vi "Konversi_Case Structure.vi"() -> ()   [LabVIEW 2020]
panel:
  in  "Case":i32
  in  "stop 2":bool
  out "Fahrenheit":dbl(slide) scale=32.0..212.0
  out "Kelvin":dbl(slide) scale=273.0..373.0
  out "Reamur":dbl(slide) scale=0.0..80.0
  in  "Celcius":dbl(slide) scale=0.0..100.0
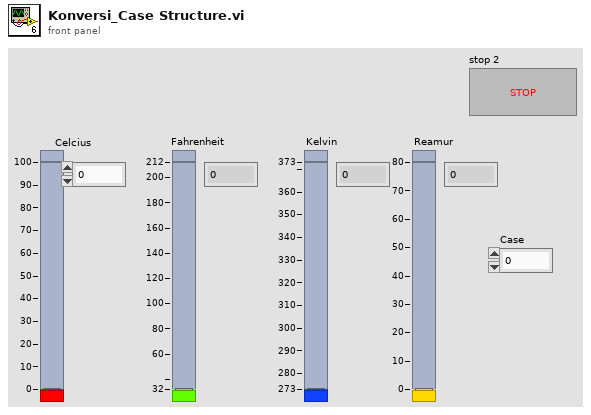
[diagram p1: front panel]
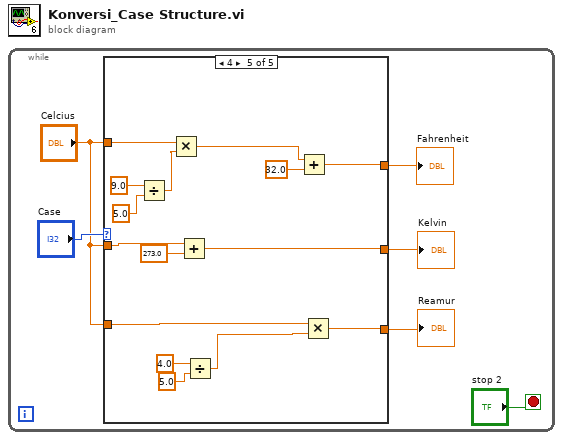
[diagram p0: block diagram]
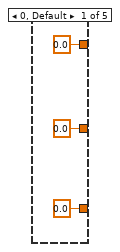
[diagram p2: hidden frame]
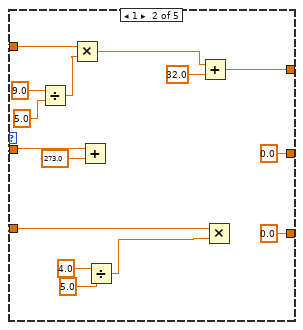
[diagram p3: hidden frame]
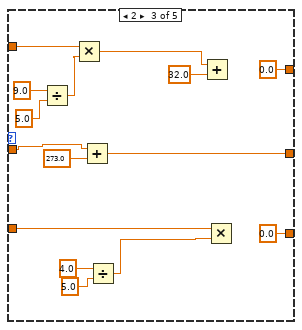
[diagram p4: hidden frame]
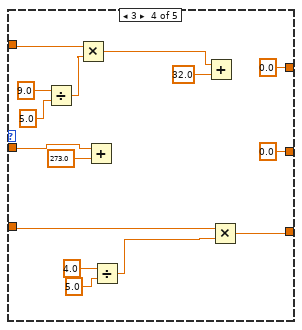
[diagram p5: hidden frame]
diagram:
  n1 = while {
    stop <- "stop 2" stop-if-true
    n2 = case shown="4" "Case" {
      tunnel: [0.0 w17 0.0 0.0 w58] -> w5
      tunnel: [0.0 0.0 w26 0.0 w57] -> w4
      tunnel: "Celcius" -> [_ w15 w29 w44 w59]
      tunnel: [0.0 0.0 0.0 w42 w56] -> w3
      tunnel: "Celcius" -> [_ _ w27 w38 w54]
      tunnel: "Celcius" -> [_ _ w25 w43 w55]
      frame 0, Default {
      }
      frame 1 {
        n3 = Divide(x=9.0, y=5.0) -> (x/y=w22:dbl)
        n4 = Multiply(x=w15, y=w22) -> (x*y=w19:dbl)
        n5 = Add(x=w15, y=273.0) -> ()  [unwired: 1 out]
        n6 = Divide(x=4.0, y=5.0) -> (x/y=w14:dbl)
        n7 = Add(x=w19, y=32.0) -> (x+y=w17:dbl)
        n8 = Multiply(x=w15, y=w14) -> ()  [unwired: 1 out]
      }
      frame 2 {
        n9 = Divide(x=9.0, y=5.0) -> (x/y=w37:dbl)
        n10 = Multiply(x=w29, y=w37) -> (x*y=w34:dbl)
        n11 = Add(x=w27, y=273.0) -> (x+y=w26:dbl)
        n12 = Divide(x=4.0, y=5.0) -> (x/y=w31:dbl)
        n13 = Add(x=w34, y=32.0) -> ()  [unwired: 1 out]
        n14 = Multiply(x=w25, y=w31) -> ()  [unwired: 1 out]
      }
      frame 3 {
        n15 = Divide(x=9.0, y=5.0) -> (x/y=w52:dbl)
        n16 = Multiply(x=w44, y=w52) -> (x*y=w49:dbl)
        n17 = Add(x=w38, y=273.0) -> ()  [unwired: 1 out]
        n18 = Divide(x=4.0, y=5.0) -> (x/y=w46:dbl)
        n19 = Add(x=w49, y=32.0) -> ()  [unwired: 1 out]
        n20 = Multiply(x=w43, y=w46) -> (x*y=w42:dbl)
      }
      frame 4 {
        n21 = Divide(x=9.0, y=5.0) -> (x/y=w67:dbl)
        n22 = Multiply(x=w59, y=w67) -> (x*y=w64:dbl)
        n23 = Add(x=w54, y=273.0) -> (x+y=w57:dbl)
        n24 = Divide(x=4.0, y=5.0) -> (x/y=w61:dbl)
        n25 = Add(x=w64, y=32.0) -> (x+y=w58:dbl)
        n26 = Multiply(x=w55, y=w61) -> (x*y=w56:dbl)
      }
    }
    "Fahrenheit" <- w5
    "Kelvin" <- w4
    "Reamur" <- w3
  }
